vi "PID_Monitor_HostGUI_DataLog.vi"() -> ()   [LabVIEW 2017]
panel:
  in  "DataLog Enable":bool
  out "Active":bool
  in  "Setpoint":dbl(slide)=50.0 scale=0.0..100.0
  out "Output (MV)":dbl(graph)
  out "HL":bool
  out "LL":bool
  in  "Max":dbl(slide)=75.0 scale=0.0..100.0
  in  "Min":dbl(slide)=25.0 scale=0.0..100.0
  out "SP":dbl(knob) scale=0.0..100.0
  out "PV":dbl(knob) scale=0.0..100.0
  out "Monitor Chart":T1(graph)
  in  "stop":bool
  # "PID Control Real-Time Demo"
  # "Press Stop for Exit"
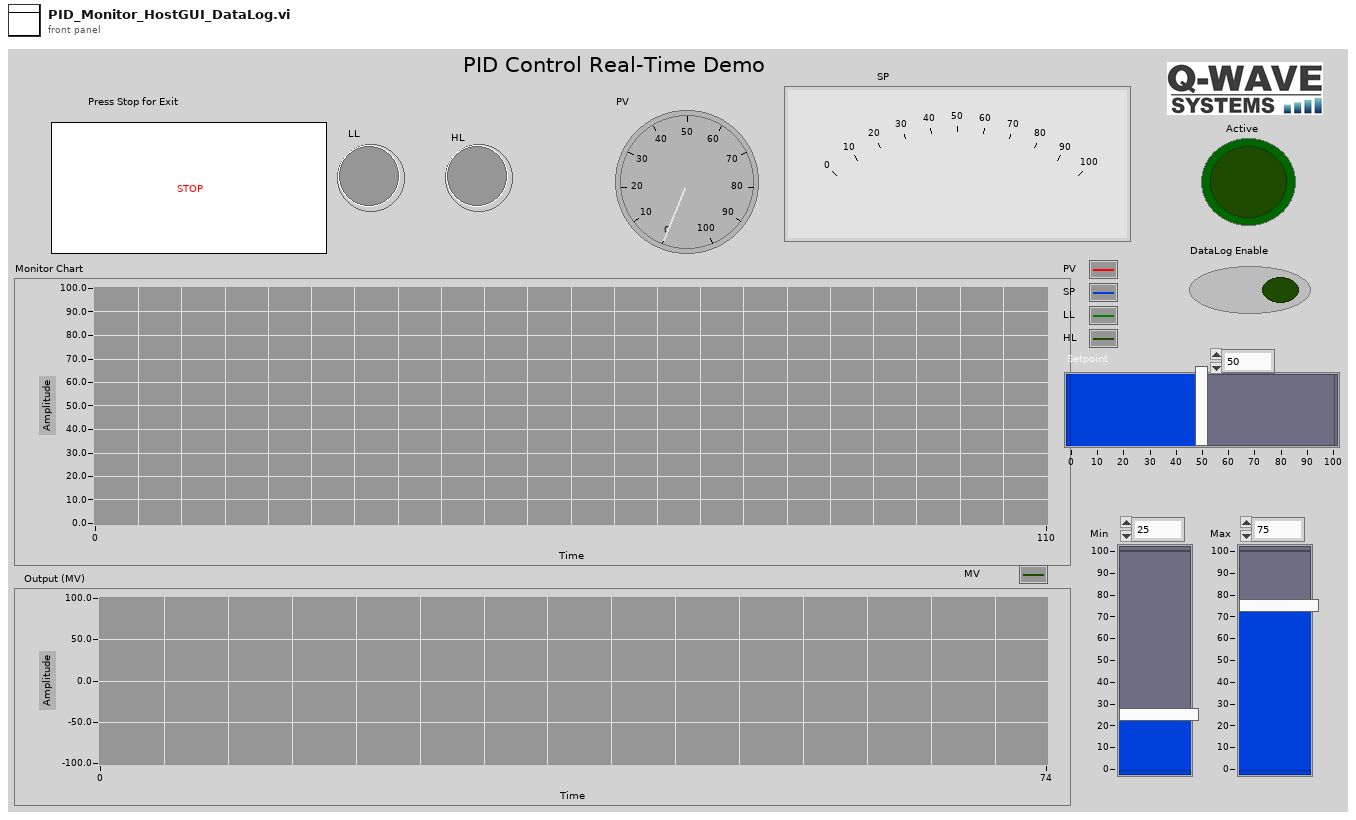
[diagram p1: front panel]
types:
  T1 = cluster{"PV":dbl, "SP":dbl, "Min":dbl, "Max":dbl}
  T2 = cluster{"Double":dbl, "Setpoint":dbl, "Min":dbl, "Max":dbl}
  T3 = enum32{"invalid app kind", "Development System", "Run Time System", "Student Edition", "Embedded LabVIEW", "Evaluation", "Custom"}
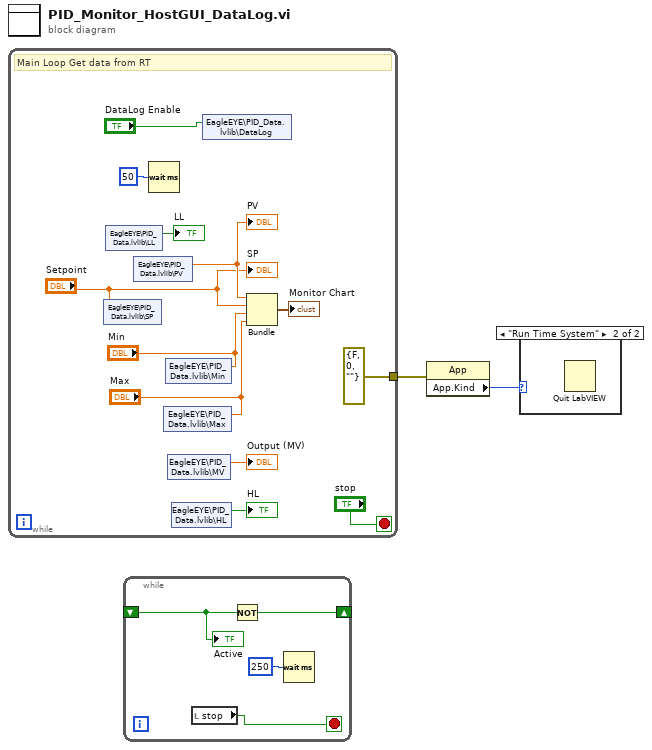
[diagram p0: block diagram]
diagram:
  n1 = while {
    tunnel: [errorcluster {"status"=FALSE, "code"=0, "source"=""} ("error in (no error)")] -> w2
    stop <- "stop" stop-if-true
    # "Main Loop Get data from RT"
    n2 = shared-variable "EagleEYE\\PID_Data.lvlib\\SP"("Setpoint") -> ()  [unwired: 1 in, 1 out]
    n3 = shared-variable "EagleEYE\\PID_Data.lvlib\\LL"() -> (→"LL":bool)  [unwired: 1 in, 1 out]
    n4 = shared-variable "EagleEYE\\PID_Data.lvlib\\PV"() -> (w6:dbl)  [unwired: 1 in, 1 out]
    "PV" <- w6
    n5 = Wait (ms)(milliseconds to wait=u32 50) -> ()  [unwired: 1 out]
    n6 = shared-variable "EagleEYE\\PID_Data.lvlib\\Max"("Max") -> ()  [unwired: 1 in, 1 out]
    n7 = shared-variable "EagleEYE\\PID_Data.lvlib\\Min"("Min") -> ()  [unwired: 1 in, 1 out]
    n8 = shared-variable "EagleEYE\\PID_Data.lvlib\\MV"() -> (→"Output (MV)":dbl)  [unwired: 1 in, 1 out]
    n9 = shared-variable "EagleEYE\\PID_Data.lvlib\\HL"() -> (→"HL":bool)  [unwired: 1 in, 1 out]
    n10 = shared-variable "EagleEYE\\PID_Data.lvlib\\DataLog"("DataLog Enable") -> ()  [unwired: 1 in, 1 out]
    n11 = Bundle("Double"=w6, "Setpoint"="Setpoint", "Min"="Min", "Max"="Max") -> (→"Monitor Chart":T2)  [unwired: 1 in]
    "SP" <- "Setpoint"
  }
  n12 = while {
    shift-right: [w16] -> _
    shift-left: _ -> [w17]
    stop <- w15 stop-if-true
    n13 = local read "stop"() -> (w15:bool)
    n14 = Not(x=w17) -> (.not. x?=w16:bool)
    n15 = Wait (ms)(milliseconds to wait=u32 250) -> ()  [unwired: 1 out]
    "Active" <- w17
  }
  n16 = property class="App"(error in=w2) -> ("App.Kind"=w1:T3)  [unwired: 1 in, 2 out]
  n17 = case shown="\"Run Time System\"" w1 {
    frame "invalid app kind", Default {
    }
    frame "Run Time System" {
      n18 = Quit LabVIEW() -> ()  [unwired: 1 in]
    }
  }
